vi "Config Key String To Numeric ID Double Numeric Map.vi"(7 "Section In":string, 8 "Error In":errorcluster, 9 "ID In":i64[](array[numeric]), 10 "Keys In":string[](array[string]), 11 "Ref In":T1) -> (0 "Error Out":errorcluster, 2 "Numeric Map Out":map{i64, dbl}(c390), 3 "Ref Out":T1)   [LabVIEW 2024]
uses:
  <vilib>/Utility/config.llb/Config Data RefNum.ctl
  <vilib>/Utility/config.llb/Read Key (Double).vi
  <vilib>/Utility/config.llb/NI_LVConfig.lvlib
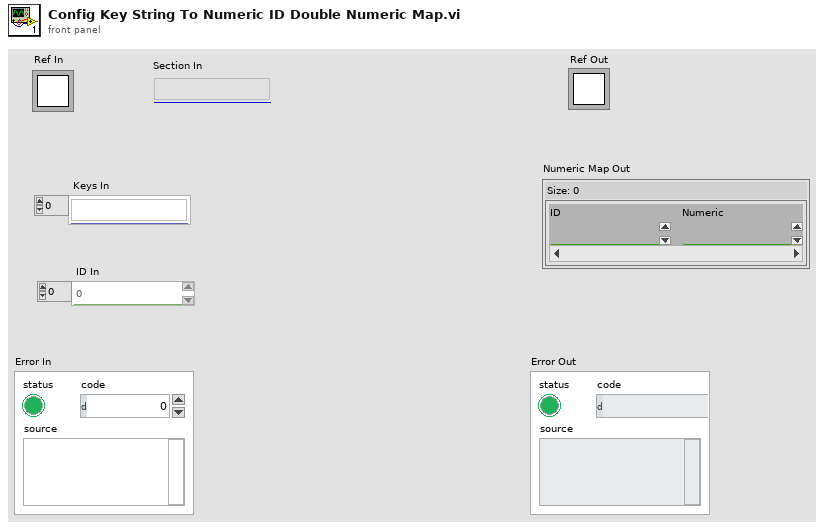
[diagram p1: front panel]
types:
  T1 = typedef "NI_LVConfig.lvlib/Config Data RefNum.ctl" = refnum<k1>
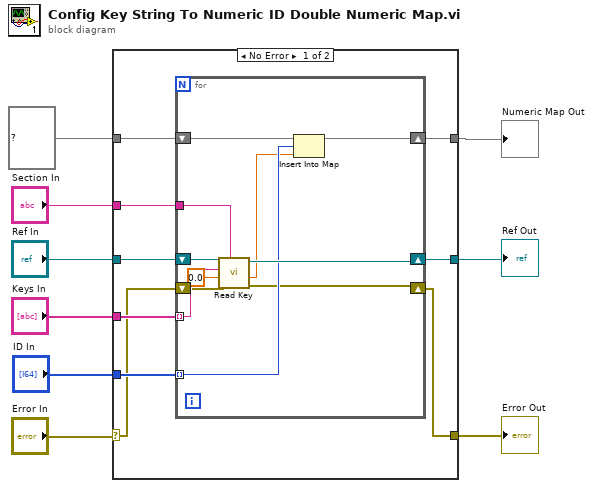
[diagram p0: block diagram]
diagram:
  n1 = case shown="No Error" "Error In" {
    selector: "Error In" -> [w12 w31]
    tunnel: "Ref In" -> [w18 w32]
    tunnel: [w17 w32] -> w8
    tunnel: "Section In" -> [w16 _]
    tunnel: [w10 w31] -> w5
    tunnel: "Keys In" -> [w15 _]
    tunnel: "ID In" -> [w14 _]
    tunnel: map{i64, dbl} {} ("Numeric Map Out") -> [w13 w30]
    tunnel: [w11 w30] -> w1
    frame No Error {
      n2 = for {
        shift-right: [w27] -> w17
        shift-left: w18 -> [w29]
        tunnel: w16 -> [w28]
        tunnel: w15 -> [w26] mode=indexing
        tunnel: w14 -> [w24] mode=indexing
        shift-right: [w20] -> w11
        shift-left: w13 -> [w25]
        shift-right: [w21] -> w10
        shift-left: w12 -> [w22]
        n3 = call-poly <vilib>:"Read Key.vi"("section"=w28, "error in (no error)"=w22, "default value"=0.0, "key"=w26, "refnum"=w29) -> ("error out"=w21:errorcluster, "value"=w23:dbl, "refnum out"=w27:T1)  [unwired: 3 in, 1 out]
        n4 = Insert Into Map(map in=w25, key=w24, value=w23) -> (map out=w20:map{i64, dbl})  [unwired: 2 out]
      }
    }
    frame Error {
    }
  }
  "Ref Out" <- w8
  "Error Out" <- w5
  "Numeric Map Out" <- w1
